vi "Register Event.vi"(8 "error in (no error)":errorcluster, 11 "Messaging in":refnum<class "Messaging.lvclass">) -> (0 "error out":errorcluster, 3 "Messaging out":refnum<class "Messaging.lvclass">)   [LabVIEW 2023, in "Messaging.lvclass"]
uses:
  Messaging.lvclass
  Messaging.lvclass/Messaging.ctl
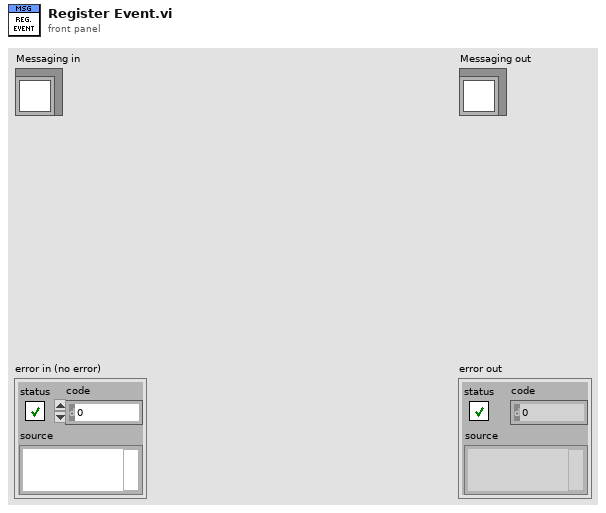
[diagram p1: front panel]
types:
  T1 = typedef "Msg.Event.Ref.ctl" = refnum<user-event>
  T2 = typedef "Msg.Event.RegRef.ctl" = refnum<event-registration>
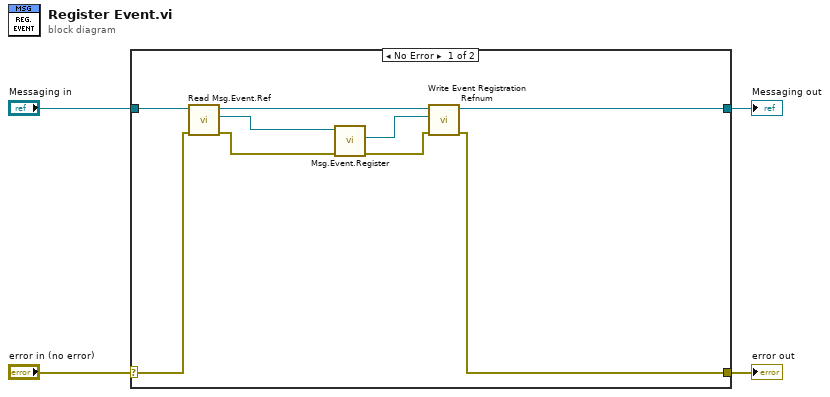
[diagram p0: block diagram]
diagram:
  n1 = case shown="No Error" "error in (no error)" {
    selector: "error in (no error)" -> [w12 w15]
    tunnel: [w7 w15] -> w3
    tunnel: [w8 w14] -> w1
    tunnel: "Messaging in" -> [w13 w14]
    frame No Error {
      n2 = call-dynamic "Read Msg.Event.Ref.vi"("error in (no error)"=w12, "Messaging in"=w13) -> ("error out"=w10:errorcluster, "Msg.Event.Ref"=w11:T1, "Messaging out"=w9:refnum<class "Messaging.lvclass">)  [unwired: 7 in]
      n3 = call "Msg.Event.Register.vi"("Error (in)"=w10, "Msg.Event.Ref"=w11) -> ("Error (out)"=w5:errorcluster, "Event Registration Refnum"=w6:T2)  [unwired: 7 in, 1 out]
      n4 = call-dynamic "Write Event Registration Refnum.vi"("error in (no error)"=w5, "Event Registration Refnum"=w6, "Messaging in"=w9) -> ("error out"=w7:errorcluster, "Messaging out"=w8:refnum<class "Messaging.lvclass">)  [unwired: 7 in]
    }
    frame Error {
    }
  }
  "error out" <- w3
  "Messaging out" <- w1
